vi "iWorx - Circulation Lab2.vi"() -> ()   [LabVIEW 2014]
uses:
  vi.lib/iWorx/iWorx Set Points.ctl
  <vilib>/DAQmx/create/channels.llb/DAQmx Create Channel (AI-Voltage-Basic).vi
  <vilib>/DAQmx/configure/timing.llb/DAQmx Timing (Sample Clock).vi
  <vilib>/DAQmx/read.llb/DAQmx Read (Analog 1D Wfm NChan NSamp).vi
  <vilib>/measure/macond.llb/IIR Filter for 1 Chan.vi
  <vilib>/measure/NI_MAPro.lvlib
panel:
  in  "Rescale Heart":bool
  in  "Reset Default Cal":bool
  in  "Set Points":T1={"SP1 Voltage"=1.79, "SP1 Value"=40.0, "SP2 Voltage"=2.18, "SP2 Value"=200.0} {"SP2 Value" format="%.1f mmHg"; "SP2 Voltage" format="%.2f V"; "SP1 Value" format="%.1f mmHg"; "SP1 Voltage" format="%.2f V"}
  out "Offset(b)":dbl=-694.3589743589741
  out "Slope(m)":dbl=410.2564102564101
  in  "Analyze":bool caption="Clear Chart"
  in  "Stop":bool
  in  "Log Info Button":bool
  out "Blood Pressure":dbl(knob) scale=0.0..200.0
  out "Blood Pressure Raw Signal":dbl format="%.3g"
  out "Pulse Chart":waveform(dbl)[](graph)
  out "Avg. Pulse":dbl format="%5.1f BPM"
  out "Inst. Pulse":dbl format="%5.1f BPM"
  in  "Threshold":dbl=0.0005 format="%_3p"
  in  "Calibrate":bool
  out "error out":errorcluster
  in  "Set Up":bool
  in  "Pause Button":bool
  in  "Snapshot Pulse":bool
  in  "Clear Charts":bool caption="Clear Chart"
  in  "Open Log Pulse":bool
  in  "Rescale Pulse":bool
  out "Pulse Raw Signal":dbl(knob) scale=-10.0..10.0
  # "Circulation Lab"
  # "Channel 1 - Pulse"
  # "Channel 2 - Blood Pressure"
  # "(            ,              )"
  # "(            ,              )"
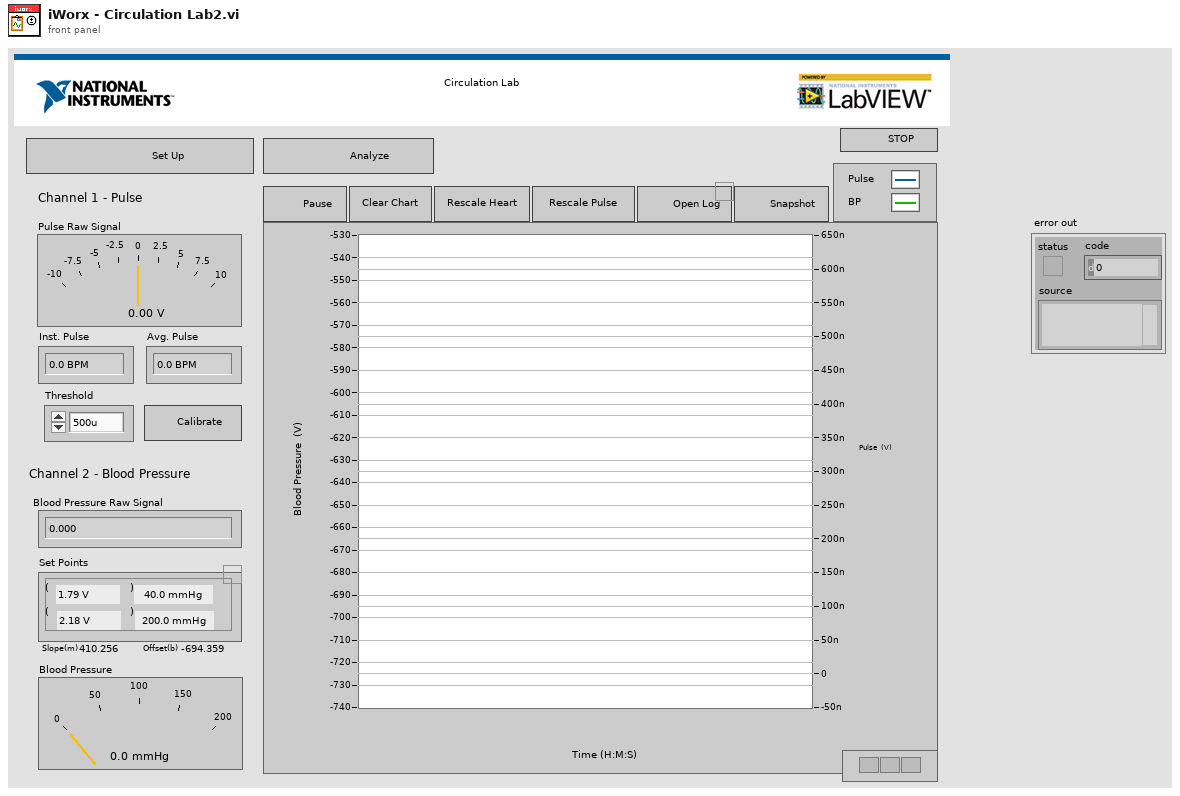
[diagram p1: front panel]
types:
  T1 = typedef "iWorx Set Points.ctl" = cluster{"SP1 Voltage":dbl, "SP1 Value":dbl, "SP2 Voltage":dbl, "SP2 Value":dbl}
  T2 = cluster{"Topology":enum16{"Off", "Butterworth", "Chebyshev", "Inverse Chebyshev", "Elliptic", "Bessel"}, "Type":enum16{"Lowpass", "Highpass", "Bandpass", "Bandstop"}, "Order":i32, "Lower Fc":dbl, "Upper Fc":dbl, "PB Ripple":dbl, "SB Attenuation":dbl}
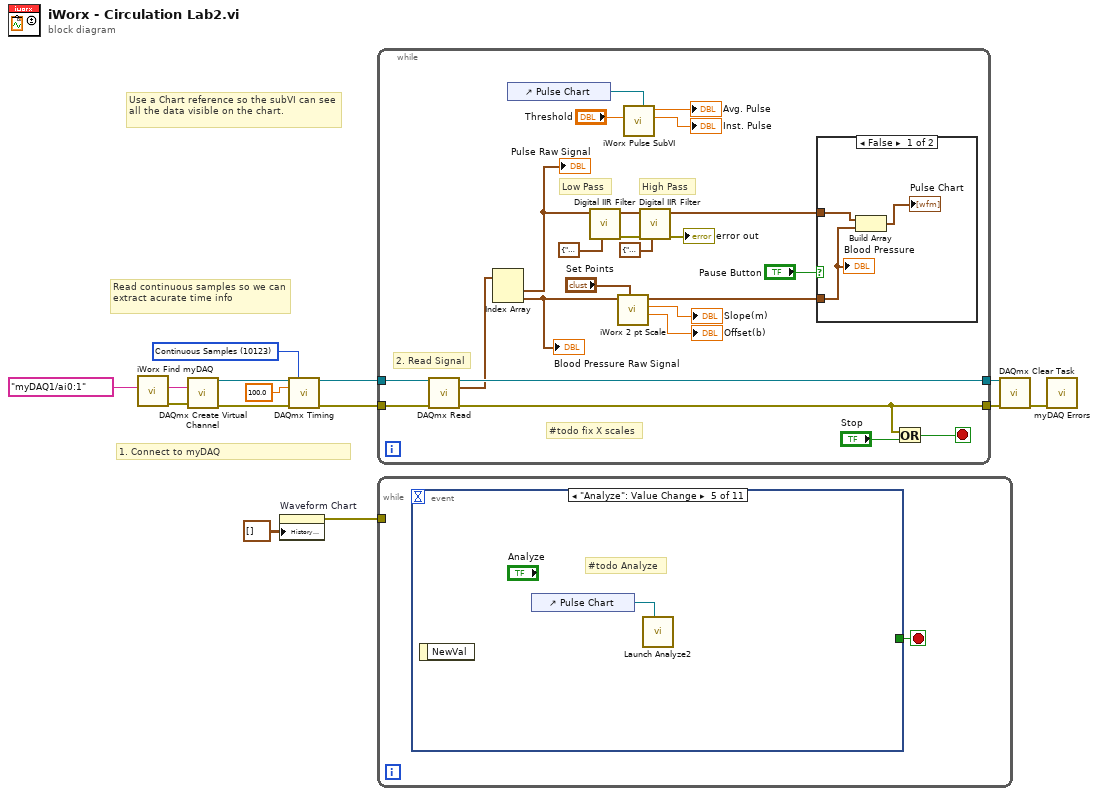
[diagram p0: block diagram]
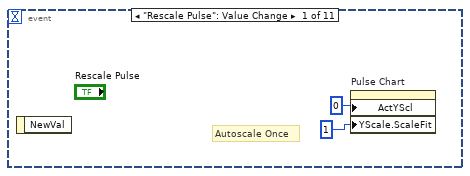
[diagram p2: hidden frame]
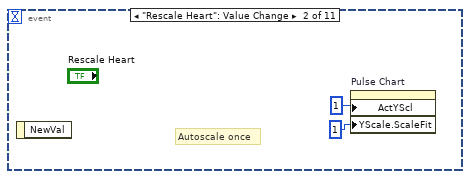
[diagram p3: hidden frame]
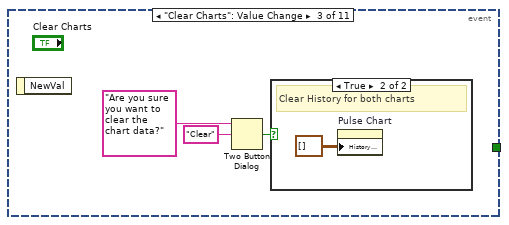
[diagram p4: hidden frame]
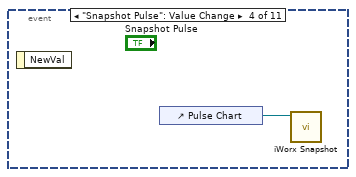
[diagram p6: hidden frame]
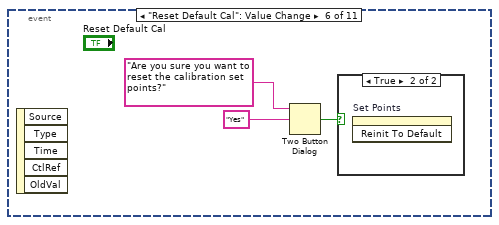
[diagram p7: hidden frame]
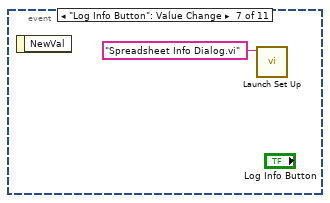
[diagram p9: hidden frame]
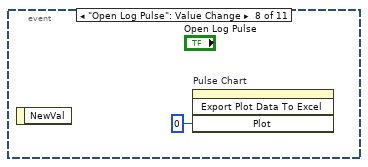
[diagram p10: hidden frame]
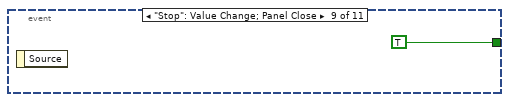
[diagram p11: hidden frame]
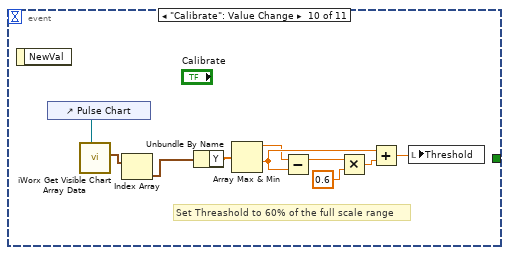
[diagram p12: hidden frame]
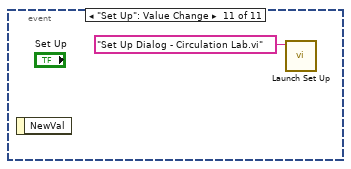
[diagram p13: hidden frame]
diagram:
  w7 = 10123 items=["Finite Samples"=10178, "Continuous Samples"=10123, "Hardware Timed Single Point"=12522] ("sample mode")
  # "1. Connect to myDAQ"
  # "Use a Chart reference so the subVI can see all the data visible on the chart."
  # "Read continuous samples so we can extract acurate time info"
  n1 = call "iWorx Find myDAQ.vi"("Preferred myDAQ (myDAQ1)"=tag "myDAQ1/ai0:1" ("physical channels")) -> ("Error Out"=w3:errorcluster, "DAQmx Physical Channel"=w4:tag)  [unwired: 6 in, 3 out]
  n2 = call-poly <vilib>:"DAQmx Create Virtual Channel.vi"("physical channels"=w4, "error in"=w3) -> ("task out"=w11:refnum<k21>, "error out"=w10:errorcluster)  [unwired: 12 in]
  n3 = property on="Waveform Chart" class="WFChart (strict)"("History Data"=waveform(dbl)[][] []) -> (error out=w12:errorcluster)  [unwired: 2 in, 1 out]
  n4 = call-poly <vilib>:"DAQmx Timing.vi"("task/channels in"=w11, "sample mode"=w7, "rate"=100.0, "error in"=w10) -> ("task out"=w8:refnum<k21>, "error out"=w9:errorcluster)  [unwired: 10 in]
  n5 = while {
    tunnel: w8 -> [w38]
    tunnel: [w37] -> w14
    tunnel: w9 -> [w36]
    tunnel: [w34] -> w13
    stop <- w35 stop-if-true
    # "#todo fix X scales"
    # "2. Read Signal"
    # "High Pass"
    # "Low Pass"
    n6 = call-poly <vilib>:"DAQmx Read.vi"("task/channels in"=w38, "error in"=w36) -> ("task out"=w37:refnum<k21>, "data"=w33:waveform(dbl)[], "error out"=w34:errorcluster)  [unwired: 11 in]
    n7 = Index Array(array=w33) -> (element #1=w26:waveform(dbl), element #2=w24:waveform(dbl))  [unwired: 2 in]
    "Pulse Raw Signal" <- w26
    "Blood Pressure Raw Signal" <- w24
    n8 = control-ref of="Pulse Chart"() -> (w15:refnum<vi>)
    n9 = call-poly <vilib>:"Digital IIR Filter.vi"("IIR filter specifications"=T2 {"Topology"=enum."Butterworth", "Type"=enum."Lowpass", "Order"=1, "Lower Fc"=0.001, "Upper Fc"=200.0, "PB Ripple"=1.0, "SB Attenuation"=60.0}, "signal in"=w26) -> ("error out"=w30:errorcluster, "signal out"=w27:waveform(dbl))  [unwired: 7 in, 1 out]
    n10 = call "iWorx 2 pt Scale.vi"("Set Points"="Set Points", "Raw Waveform"=w24) -> ("Offset"=→"Offset(b)":dbl, "Slope"=→"Slope(m)":dbl, "Scaled Value"=w23:waveform(dbl))  [unwired: 7 in]
    n11 = call "iWorx Pulse SubVI.vi"("Waveform Array Chart"=w15, "Threshold (.5mV)"="Threshold") -> ("Inst Pulse Rate (BPM)"=→"Inst. Pulse":dbl, "Average Pulse Rate (BPM)"=→"Avg. Pulse":dbl)  [unwired: 7 in, 1 out]
    n12 = call-poly <vilib>:"Digital IIR Filter.vi"("IIR filter specifications"=T2 {"Topology"=enum."Butterworth", "Type"=enum."Highpass", "Order"=1, "Lower Fc"=1.0, "Upper Fc"=10.0, "PB Ripple"=1.0, "SB Attenuation"=60.0} ("IIR filter specifications 2"), "error in (no error)"=w30, "signal in"=w27) -> ("error out"=→"error out":errorcluster, "signal out"=w29:waveform(dbl))  [unwired: 6 in, 1 out]
    n13 = case shown="False" "Pause Button" {
      tunnel: w29 -> [w41 _]
      tunnel: w23 -> [w40 _]
      frame False {
        n14 = Build Array(w41, w40) -> (→"Pulse Chart":waveform(dbl)[])
        "Blood Pressure" <- w40
      }
      frame True {
      }
    }
    n15 = Or(x=w34, y="Stop") -> (x .or. y?=w35:bool)
  }
  n16 = while {
    tunnel: w12 -> [_]
    stop <- w42 stop-if-true
    n17 = event shown="[4] \"Analyze\": Value Change" {
      selector: _ -> [_ _ _ _ _ _ _ _ _ _ _]
      dyn-events: _ -> [_ _ _ _ _ _ _ _ _ _ _]
      timeout: _ -> [_ _ _ _ _ _ _ _ _ _ _]
      tunnel: [_ _ _ _ _ _ _ _ TRUE _ _] -> w42
      event "Rescale Pulse": Value Change {
        # "Autoscale Once"
        n18 = event-data() -> ()  [unwired: 1 in, 1 out]
        n19 = property on="Pulse Chart" class="WFChart (strict)"("ActYScl"=0 ("Active Y Scale"), "YScale.ScaleFit"=u8 1 ("Y Scale.Scale Fit")) -> ()  [unwired: 2 in, 2 out]
      }
      event "Rescale Heart": Value Change {
        # "Autoscale once"
        n20 = event-data() -> ()  [unwired: 1 in, 1 out]
        n21 = property on="Pulse Chart" class="WFChart (strict)"("ActYScl"=1 ("Active Y Scale"), "YScale.ScaleFit"=u8 1 ("Y Scale.Scale Fit")) -> ()  [unwired: 2 in, 2 out]
      }
      event "Clear Charts": Value Change {
        n22 = event-data() -> ()  [unwired: 1 in, 1 out]
        n23 = Two Button Dialog(message="Are you sure you want to clear the chart data?", 2:"Clear" ("T button name (\"OK\")")) -> (T button?=w48:bool)  [unwired: 1 in]
        n24 = case shown="True" w48 {
          frame False {
            # "Dialog canceled"
          }
          frame True {
            # "Clear History for both charts"
            n25 = property on="Pulse Chart" class="WFChart (strict)"("History Data"=waveform(dbl)[][] []) -> ()  [unwired: 2 in, 2 out]
          }
        }
      }
      event "Snapshot Pulse": Value Change {
        n26 = event-data() -> ()  [unwired: 1 in, 1 out]
        n27 = control-ref of="Pulse Chart"() -> (w51:refnum<vi>)
        n28 = call "iWorx Snapshot.vi"("WaveformChart in"=w51) -> ()  [unwired: 10 in, 1 out]
      }
      event "Analyze": Value Change {
        # "#todo Analyze"
        n29 = event-data() -> ()  [unwired: 1 in, 1 out]
        n30 = control-ref of="Pulse Chart"() -> (w52:refnum<vi>)
        n31 = call "Launch Analyze2.vi"("Waveform Array Chart Ref"=w52) -> ()  [unwired: 9 in, 2 out]
      }
      event "Reset Default Cal": Value Change {
        n32 = event-data() -> ()  [unwired: 1 in, 5 out]
        n33 = Two Button Dialog(message="Are you sure you want to reset the calibration set points?", 2:"Yes" ("T button name (\"OK\")")) -> (T button?=w55:bool)  [unwired: 1 in]
        n34 = case shown="True" w55 {
          frame False {
          }
          frame True {
            n35 = invoke on="Set Points" class="Clust (strict)" method="Reinit To Default"() -> ()  [unwired: 3 in, 3 out]
          }
        }
      }
      event "Log Info Button": Value Change {
        n36 = event-data() -> ()  [unwired: 1 in, 1 out]
        n37 = call "Launch Set Up.vi"("name or relative path"="Spreadsheet Info Dialog.vi") -> ()  [unwired: 9 in, 2 out]
      }
      event "Open Log Pulse": Value Change {
        n38 = event-data() -> ()  [unwired: 1 in, 1 out]
        n39 = invoke on="Pulse Chart" class="WFChart (strict)" method="Export Plot Data To Excel"("Plot"=0) -> ()  [unwired: 3 in, 4 out]
      }
      event "Stop": Value Change; Panel Close {
        n40 = event-data() -> ()  [unwired: 1 in, 1 out]
      }
      event "Calibrate": Value Change {
        # "Set Threashold to 60% of the full scale range"
        n41 = event-data() -> ()  [unwired: 1 in, 1 out]
        n42 = control-ref of="Pulse Chart"() -> (w61:refnum<vi>)
        n43 = call "iWorx Get Visible Chart Array Data.vi"("Waveform Chart 3"=w61) -> ("Waveforms Out"=w59:waveform(dbl)[])  [unwired: 9 in, 1 out]
        n44 = Index Array(array=w59) -> (element=w60:waveform(dbl))  [unwired: 1 in]
        n45 = Unbundle By Name(w60) -> ("Y"=w63:dbl[])
        n46 = Array Max & Min(array=w63) -> (max value=w64:dbl, min value=w68:dbl)  [unwired: 2 out]
        n47 = Subtract(x=w64, y=w68) -> (x-y=w65:dbl)
        n48 = Multiply(x=w65, y=0.6) -> (x*y=w67:dbl)
        n49 = Add(x=w68, y=w67) -> (x+y=w62:dbl)
        n50 = local write "Threshold"(w62) -> ()
      }
      event "Set Up": Value Change {
        n51 = event-data() -> ()  [unwired: 1 in, 1 out]
        n52 = call "Launch Set Up.vi"("name or relative path"="Set Up Dialog - Circulation Lab.vi") -> ()  [unwired: 9 in, 2 out]
      }
    }
  }
  n53 = call <vilib>:"DAQmx Clear Task.vi"("task in"=w14, "error in"=w13) -> ("error out"=w1:errorcluster)  [unwired: 13 in]
  n54 = call "myDAQ Errors.vi"("error in (no error)"=w1) -> ()  [unwired: 10 in, 1 out]
